vi "assemble_and_save_DB.vi"(1 "error in (no error)":errorcluster, 2 "Run Info Cluster In":T1={"Set Point (*C)"=0, "Field (uT)"=0.0, "Soak Time (min)"=30, "Field on/off"=FALSE, "Atmosphere"="1", "Use DB"=enum."DB Yes", "User ID"="", "Batch / Boat ID"="", "User"="", "Note"="", "Field on (C)"=0.0, "Field off (C)"=0.0, "email address"="", "Control ramp"=FALSE, "Ramp rate"=1.0, "Contact Me"=enum."E-mail", "Test e-mail"=FALSE, "Cellular Provider"=""} {"Ramp rate" min=1.0 max=100.0}, 3 "Datafile blob":string, 4 "filename":refnum<file>) -> (0 "error out":errorcluster)   [LabVIEW 2009]
uses:
  Time_globals.vi
  <vilib>/addons/database/NI_Database_API.lvlib
panel:
  # "Run Information"
  # "(deg/min)"
  # "E-mail or text me when done at:"
  # "(enter e-mail address or phone number)"
  # "User Information"
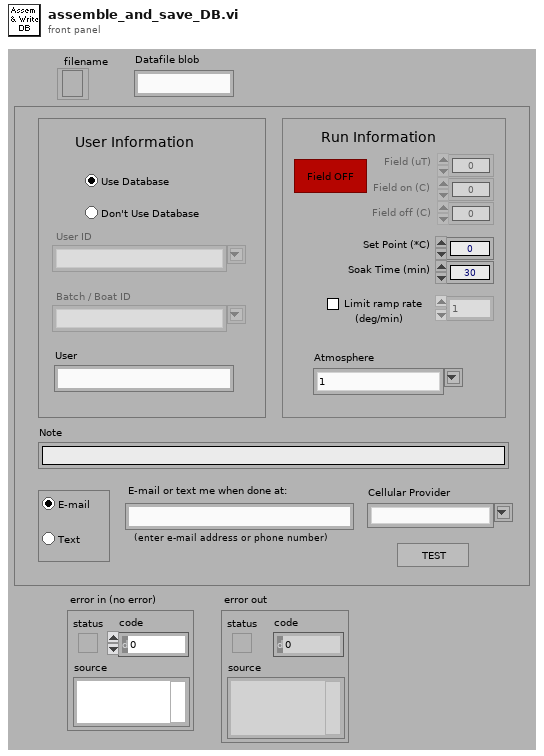
[diagram p1: front panel]
types:
  T1 = cluster{"Set Point (*C)":u32, "Field (uT)":dbl, "Soak Time (min)":u32, "Field on/off":bool, "Atmosphere":string, "Use DB":enum32{"DB Yes", "DB no"}, "User ID":string, "Batch / Boat ID":string, "User":string, "Note":string, "Field on (C)":dbl, "Field off (C)":dbl, "email address":string, "Control ramp":bool, "Ramp rate":dbl, "Contact Me":enum32{"No Selection", "E-mail", "Text"}, "Test e-mail":bool, "Cellular Provider":string}
  T2 = cluster{"User ID":string, "Batch / Boat ID":string, u32, dbl, i32, dbl, dbl, "date/time string":string, "date/time string":string, string, "Datafile blob":string}
  T3 = cluster{"User ID":string, "Batch / Boat ID":string, u32, dbl, i32, dbl, dbl, "date/time string":string, "date/time string":string, string, "Datafile blob":string, dbl, dbl}
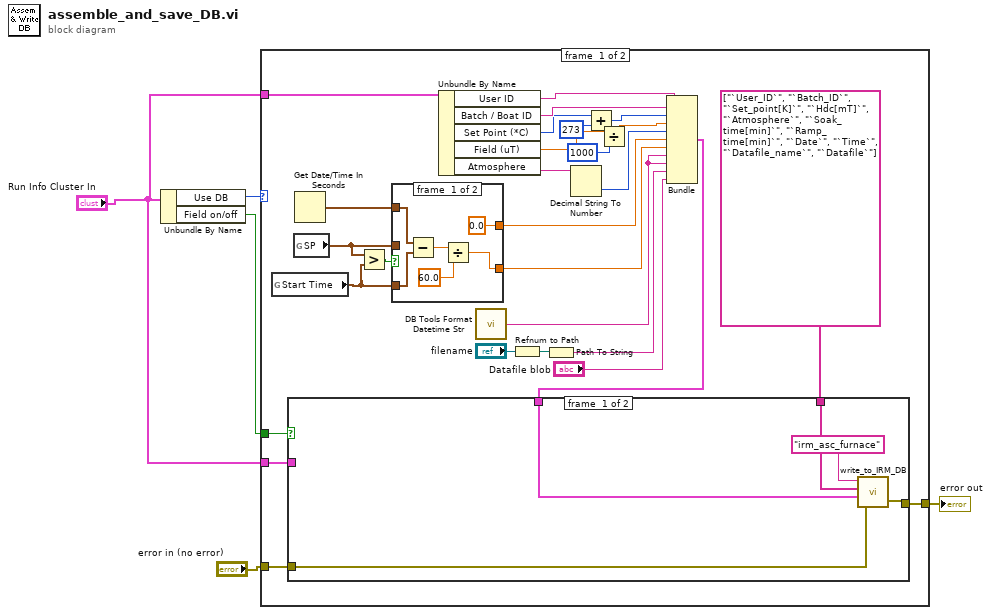
[diagram p0: block diagram]
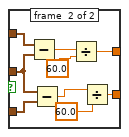
[diagram p2: hidden frame]
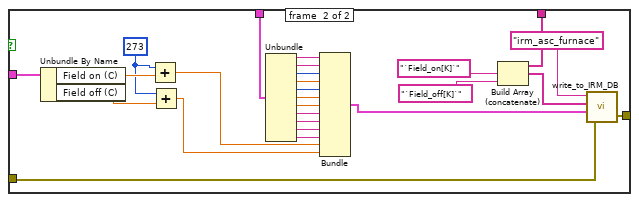
[diagram p3: hidden frame]
diagram:
  n1 = Unbundle By Name("Run Info Cluster In") -> ("Use DB"=w5:enum32{"DB Yes", "DB no"}, "Field on/off"=w4:bool)
  n2 = case shown="\"DB Yes\", Default" w5 {
    tunnel: "Run Info Cluster In" -> [w33 _]
    tunnel: w4 -> [w23 _]
    tunnel: "Run Info Cluster In" -> [w22 _]
    tunnel: "error in (no error)" -> [w14 w80]
    tunnel: [w13 w80] -> w2
    frame #0 {
      n3 = global read "Time_globals.vi" "Start Time"() -> (w7:timestamp)
      n4 = global read "Time_globals.vi" "SP"() -> (w8:timestamp)
      n5 = Get Date/Time In Seconds() -> (seconds since 1Jan1904=w11:timestamp)
      n6 = Greater?(x=w8, y=w7) -> (0:w12:bool)
      n7 = case shown="False" w12 {
        tunnel: w11 -> [w38 w46]
        tunnel: w8 -> [_ w44]
        tunnel: [0.0 w45] -> w10
        tunnel: w7 -> [w37 w43]
        tunnel: [w34 w40] -> w9
        frame #0 {
          n8 = Subtract(x=w38, y=w37) -> (x-y=w36:dbl)
          n9 = Divide(x=w36, y=60.0) -> (x/y=w34:dbl)
        }
        frame #1 {
          n10 = Subtract(x=w46, y=w44) -> (x-y=w47:dbl)
          n11 = Subtract(x=w44, y=w43) -> (x-y=w42:dbl)
          n12 = Divide(x=w47, y=60.0) -> (x/y=w45:dbl)
          n13 = Divide(x=w42, y=60.0) -> (x/y=w40:dbl)
        }
      }
      n14 = Unbundle By Name(w33) -> ("User ID"=w32:string, "Batch / Boat ID"=w31:string, "Set Point (*C)"=w21:u32, "Field (uT)"=w17:dbl, "Atmosphere"=w30:string)
      n15 = call <vilib>:"DB Tools Format Datetime Str.vi"() -> ("date/time string"=w28:string)  [unwired: 1 in]
      n16 = Refnum to Path(1:"filename") -> (0:w26:path)
      n17 = Path To String(path=w26) -> (string=w25:string)
      n18 = Decimal String To Number(string=w30) -> (number=w29:i32)  [unwired: 3 out]
      n19 = Add(x=w21, y=273) -> (x+y=w19:u32)
      n20 = Divide(x=w17, y=1000) -> (x/y=w16:dbl)
      n21 = Bundle("User ID"=w32, "Batch / Boat ID"=w31, w19, w16, w29, w10, w9, "date/time string"=w28, "date/time string"=w28, w25, "Datafile blob"="Datafile blob") -> (w6:T2)  [unwired: 1 out]
      n22 = case shown="True" w23 {
        tunnel: w22 -> [_ w79]
        tunnel: string[] ["`User_ID`", "`Batch_ID`", "`Set_point[K]`", "`Hdc[mT]`", "`Atmosphere`", "`Soak_time[min]`", "`Ramp_time[min]`", "`Date`", "`Time`", "`Datafile_name`", "`Datafile`"] -> [w52 w75]
        tunnel: w14 -> [w51 w70]
        tunnel: [w50 w69] -> w13
        tunnel: w6 -> [w49 w68]
        frame #0 {
          n23 = call "write_to_IRM_DB.vi"("error in (no error)"=w51, "data"=w49, "columns"=w52, "DB table"="irm_asc_furnace") -> ("error out"=w50:errorcluster)  [unwired: 1 out]
        }
        frame #1 {
          w76 = 273
          n24 = Unbundle By Name(w79) -> ("Field on (C)"=w78:dbl, "Field off (C)"=w77:dbl)
          n25 = Add(x=w76, y=w78) -> (x+y=w56:dbl)
          n26 = Add(x=w76, y=w77) -> (x+y=w55:dbl)
          n27 = Unbundle(w68) -> ("User ID"=w67:string, "Batch / Boat ID"=w66:string, w65:u32, w64:dbl, w63:i32, w62:dbl, w61:dbl, "date/time string"=w60:string, "date/time string"=w59:string, w58:string, "Datafile blob"=w57:string)
          n28 = Bundle("User ID"=w67, "Batch / Boat ID"=w66, w65, w64, w63, w62, w61, "date/time string"=w60, "date/time string"=w59, w58, "Datafile blob"=w57, w56, w55) -> (w54:T3)  [unwired: 1 out]
          n29 = Build Array (concatenate)(w75, "`Field_on[K]`", "`Field_off[K]`") -> (w74:string[])
          n30 = call "write_to_IRM_DB.vi"("error in (no error)"=w70, "data"=w54, "columns"=w74, "DB table"="irm_asc_furnace") -> ("error out"=w69:errorcluster)  [unwired: 1 out]
        }
      }
    }
    frame #1 {
    }
  }
  "error out" <- w2
